vi "edittest check edit permission.vi"(5 "User Information":T2, 7 "Sequence Record":T1) -> (2 "Okay to Edit?":bool)   [LabVIEW 2011]
uses:
  server/database/Users/User Record.ctl
  server/database/Sequences/Sequence Record.ctl
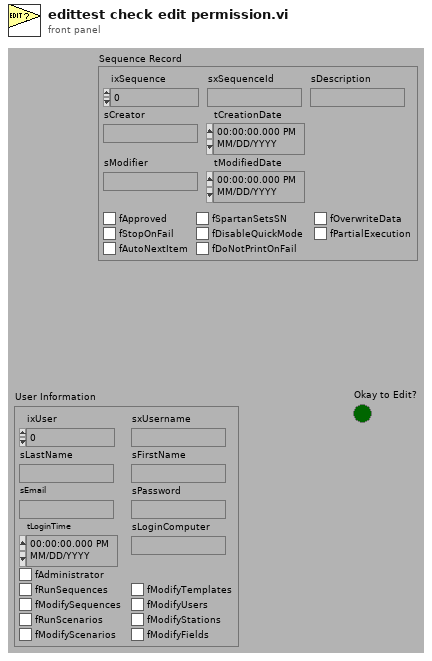
[diagram p1: front panel]
types:
  T1 = typedef "Sequence Record.ctl" = cluster{"ixSequence":i32, "sxSequenceId":string, "sDescription":string, "sCreator":string, "tCreationDate":timestamp, "sModifier":string, "tModifiedDate":timestamp, "fApproved":bool, "fSpartanSetsSN":bool, "fOverwriteData":bool, "fStopOnFail":bool, "fDisableQuickMode":bool, "fPartialExecution":bool, "fAutoNextItem":bool, "fDoNotPrintOnFail":bool}
  T2 = typedef "User Record.ctl" = cluster{"ixUser":i32, "sxUsername":string, "sLastName":string, "sFirstName":string, "sEmail":string, "sPassword":string, "tLoginTime":timestamp, "sLoginComputer":string, "fAdministrator":bool, "fRunSequences":bool, "fModifySequences":bool, "fRunScenarios":bool, "fModifyScenarios":bool, "fModifyTemplates":bool, "fModifyUsers":bool, "fModifyStations":bool, "fModifyFields":bool}
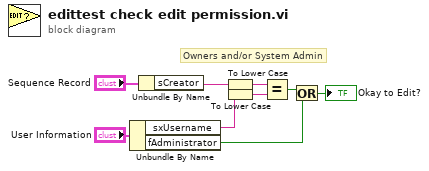
[diagram p0: block diagram]
diagram:
  # "Owners and/or System Admin"
  n1 = Unbundle By Name("User Information") -> ("sxUsername"=w7:string, "fAdministrator"=w4:bool)
  n2 = Unbundle By Name("Sequence Record") -> ("sCreator"=w8:string)
  n3 = To Lower Case(string=w8) -> (all lower case string=w9:string)
  n4 = To Lower Case(string=w7) -> (all lower case string=w6:string)
  n5 = Equal?(x=w9, y=w6) -> (x = y?=w5:bool)
  n6 = Or(x=w5, y=w4) -> (x .or. y?=→"Okay to Edit?":bool)
